vi "Temperature Warnings.vi"() -> ()   [LabVIEW 2015]
panel:
  in  "stop":bool
  out "Warning":bool
  out "Warning Text":string
  in  "Min":dbl
  in  "Max":dbl
  in  "Current Temp":dbl
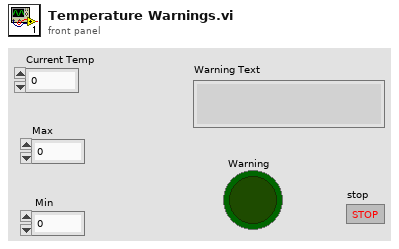
[diagram p1: front panel]
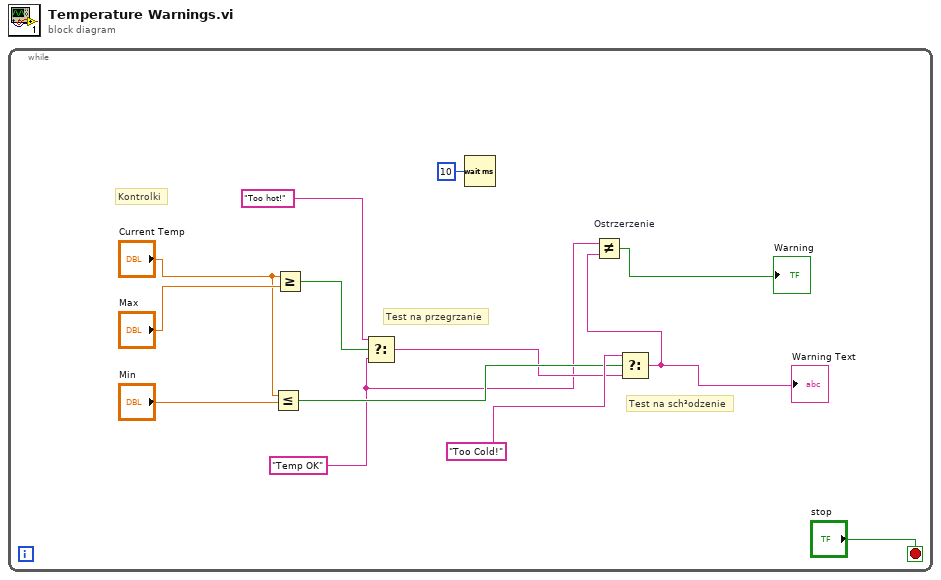
[diagram p0: block diagram]
diagram:
  n1 = while {
    stop <- "stop" stop-if-true
    w5 = "Temp OK"
    # "Test na sch³odzenie"
    # "Test na przegrzanie"
    # "Kontrolki"
    n2 = Less Or Equal?(x="Current Temp", y="Min") -> (x <= y?=w7:bool)
    n3 = Greater Or Equal?(x="Current Temp", y="Max") -> (x >= y?=w10:bool)
    n4 = Select(t="Too hot!", s=w10, f=w5) -> (s? t:f=w6:string)
    n5 = Wait (ms)(milliseconds to wait=u32 10) -> ()  [unwired: 1 out]
    n6 = Select(t="Too Cold!", s=w7, f=w6) -> (s? t:f=w3:string)
    "Warning Text" <- w3
    n7 = Not Equal? "Ostrzerzenie"(x=w5, y=w3) -> (x != y?=→"Warning":bool)
  }
